vi "ZZZ Chroma 1905x Series Start and Get Data.vi"(0 "inst handle in":refnum<visa-resource-name>, 3 "error in":T1) -> (1 "Voltage":string, 4 "Judgement Overall":string, 5 "Current":string, 6 "inst handle out":refnum<visa-resource-name>, 8 "Judgement Last Test":string, 9 "error out":T1)   [LabVIEW 2025]
doc: "Contact Chroma\nTEL: +886-2-2298-3855 \nTEL: +886-3-397-5788 \nFAX: +886-2-2298-3596\nFAX: +886-3-327-4703 \nURL: http://www.chromaate.com \nE-mail: chroma@chroma.com.tw"
uses:
  <instrlib>/Chroma 19052/Chroma 19052.lvlib
panel:
  out "number":dbl format="%.2f"
  out "Result":string
  # "Start and Get Data"
  # "Judgement\n120-121 Fail\n116   Pass\n115   Testing\n114   Cannot Test\n113   User Stop\n112   Stop\n17 - 55 Fail"
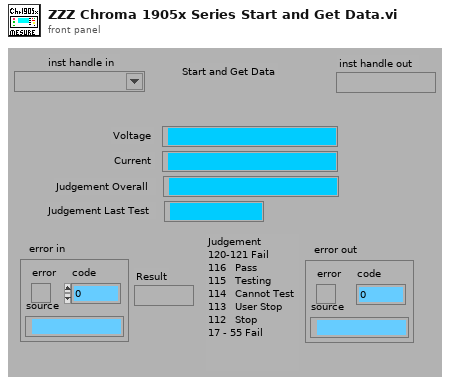
[diagram p1: front panel]
types:
  T1 = cluster{"error":bool, "code":i8, "source":string}
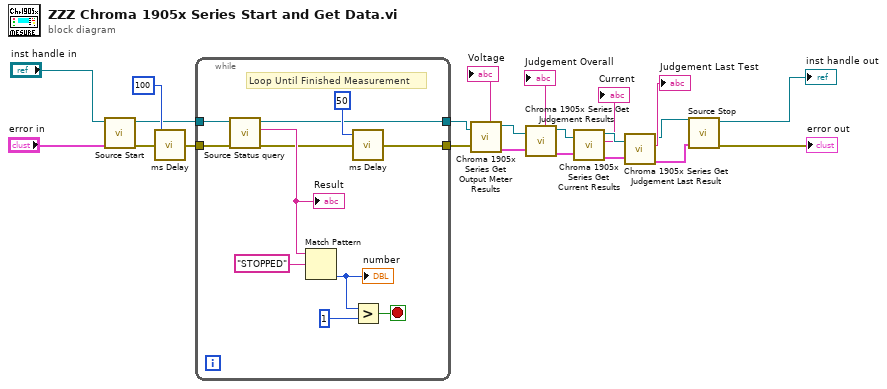
[diagram p0: block diagram]
diagram:
  n1 = call <instrlib>:"Source Start.vi"("error in (no error)"="error in", "VISA resource name"="inst handle in") -> ("error out"=w2:errorcluster, "VISA resource name out"=w1:refnum<visa-resource-name>)  [unwired: 8 in]
  n2 = call <instrlib>:"ms Delay.vi"("miliseconds to wait"=u32 100 ("Time Delay S"), "error in (no error)"=w2) -> ("error out"=w21:errorcluster)  [unwired: 6 in, 1 out]
  n3 = while {
    tunnel: [w24] -> w19
    tunnel: [w27] -> w20
    tunnel: w21 -> [w32]
    tunnel: w1 -> [w33]
    stop <- w23 stop-if-true
    # "Loop Until Finished Measurement"
    n4 = call <instrlib>:"Source Status query.vi"("error in (no error)"=w32, "VISA resource name"=w33) -> ("error out"=w25:errorcluster, "Status"=w30:string, "VISA resource name out"=w24:refnum<visa-resource-name>)  [unwired: 7 in]
    "Result" <- w30
    n5 = Match Pattern(string=w30, regular expression="STOPPED" ("format string")) -> (offset past match=w29:i32)  [unwired: 1 in, 3 out]
    "number" <- w29
    n6 = call <instrlib>:"ms Delay.vi"("miliseconds to wait"=u32 50 ("Time Delay S"), "error in (no error)"=w25) -> ("error out"=w27:errorcluster)  [unwired: 6 in, 1 out]
    n7 = Greater?(x=w29, y=1) -> (0:w23:bool)
  }
  n8 = call "Chroma 1905x Series Get Output Meter Results.vi"("inst handle Out"=w19, "error in"=w20) -> ("inst handle in"=w18:refnum<visa-resource-name>, "Result"=→"Voltage":string, "error out"=w9:T1)  [unwired: 1 in]
  n9 = call "Chroma 1905x Series Get Judgement Results.vi"("inst handle Out"=w18, "error in"=w9) -> ("inst handle in"=w16:refnum<visa-resource-name>, "Result"=→"Judgement Overall":string, "error out"=w17:T1)  [unwired: 1 in]
  n10 = call "Chroma 1905x Series Get Current Results.vi"("inst handle Out"=w16, "error in"=w17) -> ("inst handle in"=w13:refnum<visa-resource-name>, "Result"=→"Current":string, "error out"=w12:T1)  [unwired: 1 in]
  n11 = call "Chroma 1905x Series Get Judgement Last Result.vi"("inst handle Out"=w13, "error in"=w12) -> ("inst handle in"=w8:refnum<visa-resource-name>, "Result"=→"Judgement Last Test":string, "error out"=w6:T1)  [unwired: 1 in]
  n12 = call <instrlib>:"Source Stop.vi"("error in (no error)"=w6, "VISA resource name"=w8) -> ("error out"=→"error out":errorcluster, "VISA resource name out"=→"inst handle out":refnum<visa-resource-name>)  [unwired: 8 in]
